vi "ZCAN_Transmit.vi"(0 "can_index_handle":u32, 1 "Agreement":T2, 2 "fd_additional_flags":u32, 5 "can_id":u32, 7 "frame_type":T1, 9 "frame_format":i16, 11 "error in (no error)":errorcluster caption="错误输入（无错误）", 13 "Send_string_data":string) -> (15 "error out":errorcluster caption="错误输出")   [LabVIEW 2020, in "zlgcan.lvlib"]
uses:
  zlgcan.lvlib
  data_type/Agreement.ctl
  data_type/frame type.ctl
  bin/zlgcan_wrap.dll
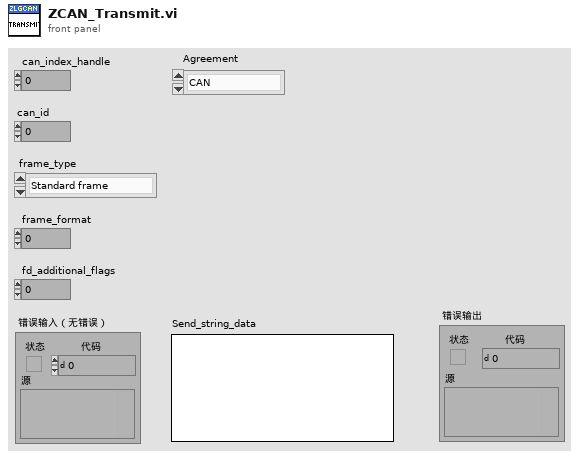
[diagram p1: front panel]
types:
  T1 = typedef "zlgcan.lvlib/frame type.ctl" = enum32{"Standard frame", "Extended frame"}
  T2 = typedef "zlgcan.lvlib/Agreement.ctl" = enum16{"CAN", "CANFD"}
  T3 = typedef "zlgcan.lvlib/tagZCAN_TransmitFD_Data.ctl" = cluster{"canfd_frame":T4, "transmit_type":u32}
  T4 = typedef "zlgcan.lvlib/canfd_frame.ctl" = cluster{"can_id":u32, "len":u8, "flags":u8, "__res0":u8, "__res1":u8, "data":cluster{"CAN数据[0]":u8, "CAN数据[1]":u8, "CAN数据[2]":u8, "CAN数据[3]":u8, "CAN数据[4]":u8, "CAN数据[5]":u8, "CAN数据[6]":u8, "CAN数据[7]":u8, "CAN数据[8]":u8, "CAN数据[9]":u8, "CAN数据[10]":u8, "CAN数据[11] ":u8, "CAN数据[12] ":u8, "CAN数据[13] ":u8, "CAN数据[14] ":u8, "CAN数据[15] ":u8, "CAN数据[16]":u8, "CAN数据[17]":u8, "CAN数据[18]":u8, "CAN数据[19]":u8, "CAN数据[20]":u8, "CAN数据[21]":u8, "CAN数据[22]":u8, "CAN数据[23]":u8, "CAN数据[24] ":u8, "CAN数据[25]":u8, "CAN数据[26]":u8, "CAN数据[27]":u8, "CAN数据[28]":u8, "CAN数据[29]":u8, "CAN数据[30]":u8, "CAN数据[31]":u8, "CAN数据[32]":u8, "CAN数据[33]":u8, "CAN数据[34]":u8, "CAN数据[35]":u8, "CAN数据[36]":u8, "CAN数据[37]":u8, "CAN数据[38]":u8, "CAN数据[39]":u8, "CAN数据[40]":u8, "CAN数据[41]":u8, "CAN数据[42]":u8, "CAN数据[43]":u8, "CAN数据[44]":u8, "CAN数据[45]":u8, "CAN数据[46]":u8, "CAN数据[47]":u8, "CAN数据[48]":u8, "CAN数据[49]":u8, "CAN数据[50]":u8, "CAN数据[51]":u8, "CAN数据[52]":u8, "CAN数据[53]":u8, "CAN数据[54]":u8, "CAN数据[55]":u8, "CAN数据[56]":u8, "CAN数据[57]":u8, "CAN数据[58]":u8, "CAN数据[59]":u8, "CAN数据[60]":u8, "CAN数据[61]":u8, "CAN数据[62]":u8, "CAN数据[63]":u8}}
  T5 = typedef "zlgcan.lvlib/tagZCAN_Transmit_Data.ctl" = cluster{"can_frame":T6, "transmit_type":u32}
  T6 = typedef "zlgcan.lvlib/can_frame.ctl" = cluster{"can_id":u32, "can_dlc":u8, "__pad":u8, "__res0":u8, "__res1":u8, "data":cluster{"CAN数据[0]":u8, "CAN数据[1]":u8, "CAN数据[2]":u8, "CAN数据[3]":u8, "CAN数据[4]":u8, "CAN数据[5]":u8, "CAN数据[6]":u8, "CAN数据[7]":u8}}
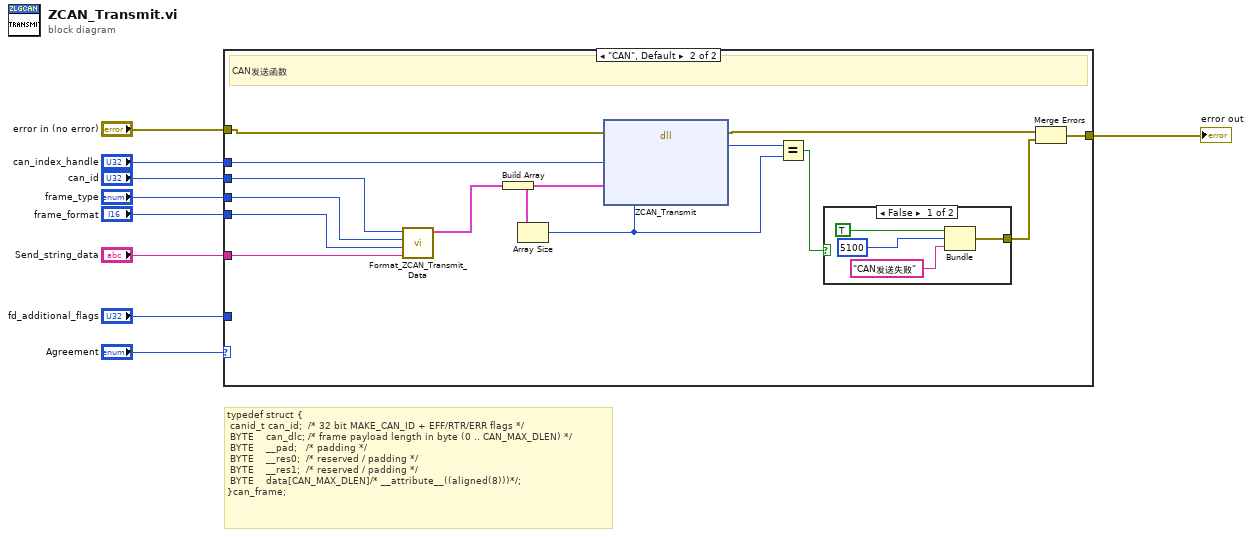
[diagram p0: block diagram]
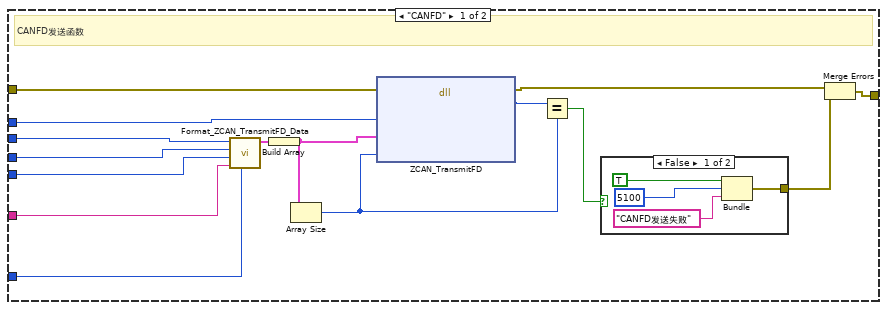
[diagram p2: hidden frame]
diagram:
  # "typedef struct {\n\tcanid_t can_id;  /* 32 bit MAKE_CAN_ID + EFF/RTR/ERR flags */\n\tBYTE    can_dlc; /* frame payload length in byte (0 .. CAN_MAX_DLEN) */\n\tBYTE    __pad;   /* padding */\n\tBYTE    __res0;  /* reserved / padding */\n\tBYTE    __res1;  /* reserved / padding */\n\tBYTE    data[CAN_MAX_DLEN]/* __attribute__((aligned(8)))*/;\n}can_frame;"
  n1 = case shown="\"CAN\", Default" "Agreement" {
    tunnel: [w11 w31] -> w9
    tunnel: "can_index_handle" -> [w15 w39]
    tunnel: "can_id" -> [w20 w38]
    tunnel: "frame_type" -> [w19 w37]
    tunnel: "frame_format" -> [w18 w36]
    tunnel: "fd_additional_flags" -> [w17 _]
    tunnel: "Send_string_data" -> [w16 w35]
    tunnel: "error in (no error)" -> [w12 w29]
    frame "CANFD" {
      # "CANFD发送函数"
      n2 = call "Format_ZCAN_TransmitFD_Data.vi"("fd_additional _flags"=w17, "Send_string_data"=w16, "frame_format"=w18, "frame_type"=w19, "can_frame.can_id"=w20) -> ("tagZCAN_TransmitFD_Data"=w21:T3)  [unwired: 6 in]
      n3 = Build Array(w21) -> (w14:T3[])
      n4 = Array Size(array=w14) -> (size(s)=w13:i32)
      n5 = dll-call lib="D:/Git/ZLG_USBCANFD/bin/zlgcan_wrap.dll" fn="ZCAN_TransmitFD"(error in=w12, "通道句柄"=w15, "数据帧数组"=w14, "数据帧数"=w13) -> (error out=w10:errorcluster, "返回类型"=w24:u32)  [unwired: 5 in, 1 out]
      n6 = Equal?(x=w24, y=w13) -> (x = y?=w23:bool)
      n7 = case shown="False" w23 {
        tunnel: [w25 _] -> w22
        frame False {
          n8 = Bundle("status"=TRUE, "code"=5100, "消息"="CANFD发送失败") -> (w25:cluster{"status":bool, "code":i32, "消息":string})  [unwired: 1 in]
        }
        frame True {
        }
      }
      n9 = Merge Errors(w10, w22) -> (w11:errorcluster)
    }
    frame "CAN", Default {
      # "CAN发送函数"
      n10 = call "Format_ZCAN_Transmit_Data.vi"("Send_string_data"=w35, "frame_format"=w36, "frame_type"=w37, "can_frame.can_id"=w38) -> ("tagZCAN_Transmit_Data"=w42:T5)  [unwired: 7 in]
      n11 = Build Array(w42) -> (w34:T5[])
      n12 = Array Size(array=w34) -> (size(s)=w33:i32)
      n13 = dll-call lib="D:/Git/ZLG_USBCANFD/bin/zlgcan_wrap.dll" fn="ZCAN_Transmit"(error in=w29, "通道句柄"=w39, "数据帧数组"=w34, "数据帧数"=w33) -> (error out=w30:errorcluster, "返回类型"=w41:u32)  [unwired: 5 in, 1 out]
      n14 = Equal?(x=w41, y=w33) -> (x = y?=w40:bool)
      n15 = case shown="False" w40 {
        tunnel: [w43 _] -> w32
        frame False {
          n16 = Bundle("status"=TRUE, "code"=5100, "消息"="CAN发送失败") -> (w43:cluster{"status":bool, "code":i32, "消息":string})  [unwired: 1 in]
        }
        frame True {
        }
      }
      n17 = Merge Errors(w30, w32) -> (w31:errorcluster)
    }
  }
  "error out" <- w9
